vi "generate 96 well rois.vi"() -> ()   [LabVIEW 2013]
uses:
  <vilib>/vision/NI_Vision_Development_Module.lvlib
panel:
  in  "Save ROI data":path=path "C:/Users/Ed/Desktop/test temo2.png"
  out "roi data cluster":T1
  in  "Options":T2={"Interpolation Type"=enum."Bilinear Fixed", "Destination Width"=0, "Destination Height"=0, "Fill Value"=0.0}
  in  "Define Corner":bool
  in  "num Y cells":dbl=8.0
  in  "num X cells":dbl=12.0
  in  "three points":dbl[][](array[numeric])=[[86.0, 147.0], [2469.0, 46.0], [2531.0, 1640.0]]
  out "Image":T3(plugin-control)
  in  "Path to Image":path=path "C:/Users/Ed/Desktop/test temo2.png"
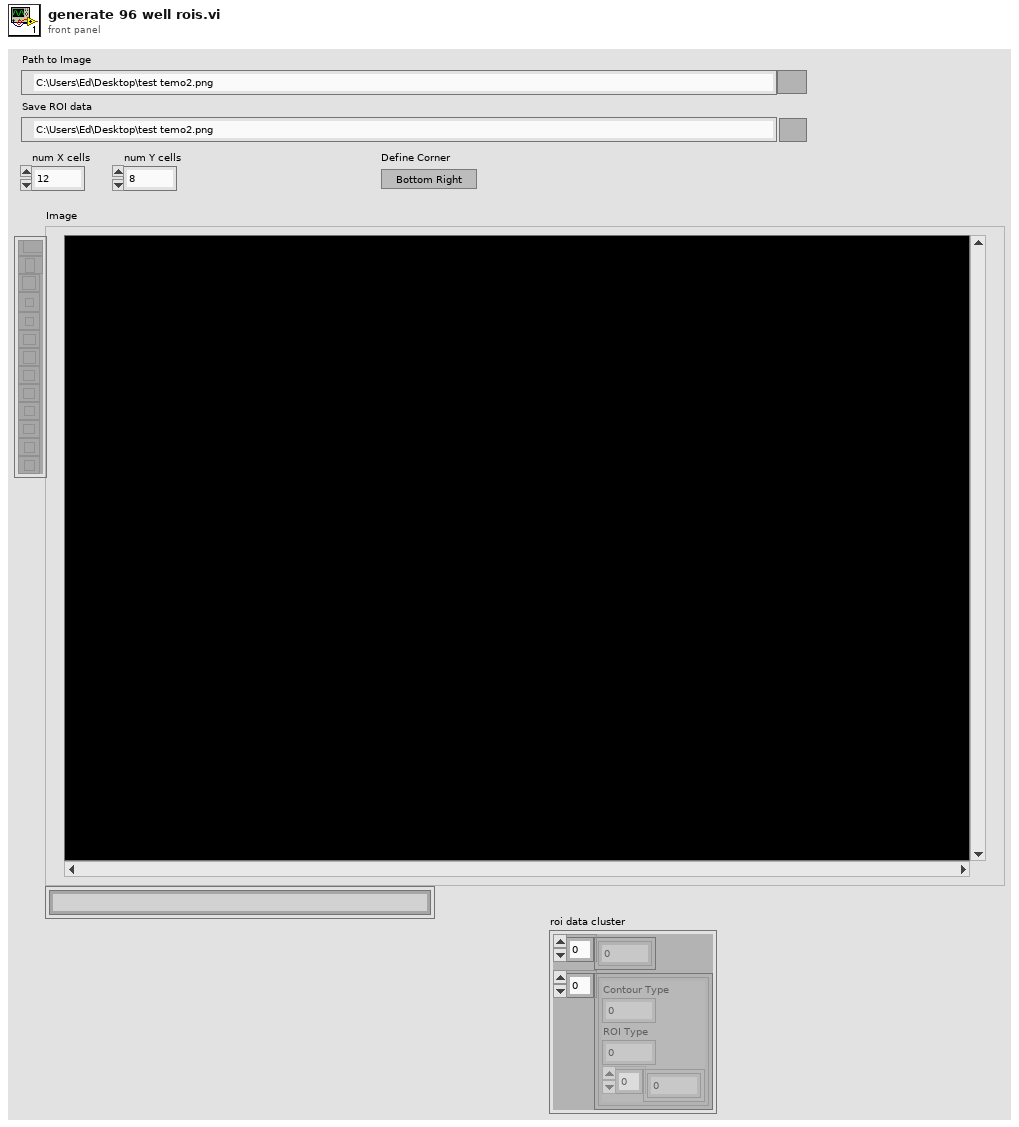
[diagram p1: front panel]
types:
  T1 = cluster{i32[], cluster{"Contour Type":u32, "ROI Type":u32, i32[]}[]}
  T2 = cluster{"Interpolation Type":enum32{"Zero Order", "Bilinear", "Quadratic", "Cubic", "Bilinear Fixed"}, "Destination Width":u32, "Destination Height":u32, "Fill Value":sgl}
  T3 = typedef "IMAQ Image.ctl" = refnum<image>
  T4 = enum16{"open", "replace", "create", "open or create", "replace or create", "replace or create with confirmation"}
  T5 = cluster{"Global Rectangle":i32[], "Contours":cluster{"Contour Type":u32, "ROI Type":u32, "Points":i32[]}[]}
  T6 = cluster{"Contour Type":u32, "ROI Type":u32, "Points":i32[]}[]
  T7 = cluster{"Contour Type":u32, "ROI Type":u32, "Points":i32[]}
  T8 = cluster{"Contour Type":u32, "ROI Type":u32, i32[]}
  T9 = cluster{"Contour Type":u32, "ROI Type":u32, i32[]}[]
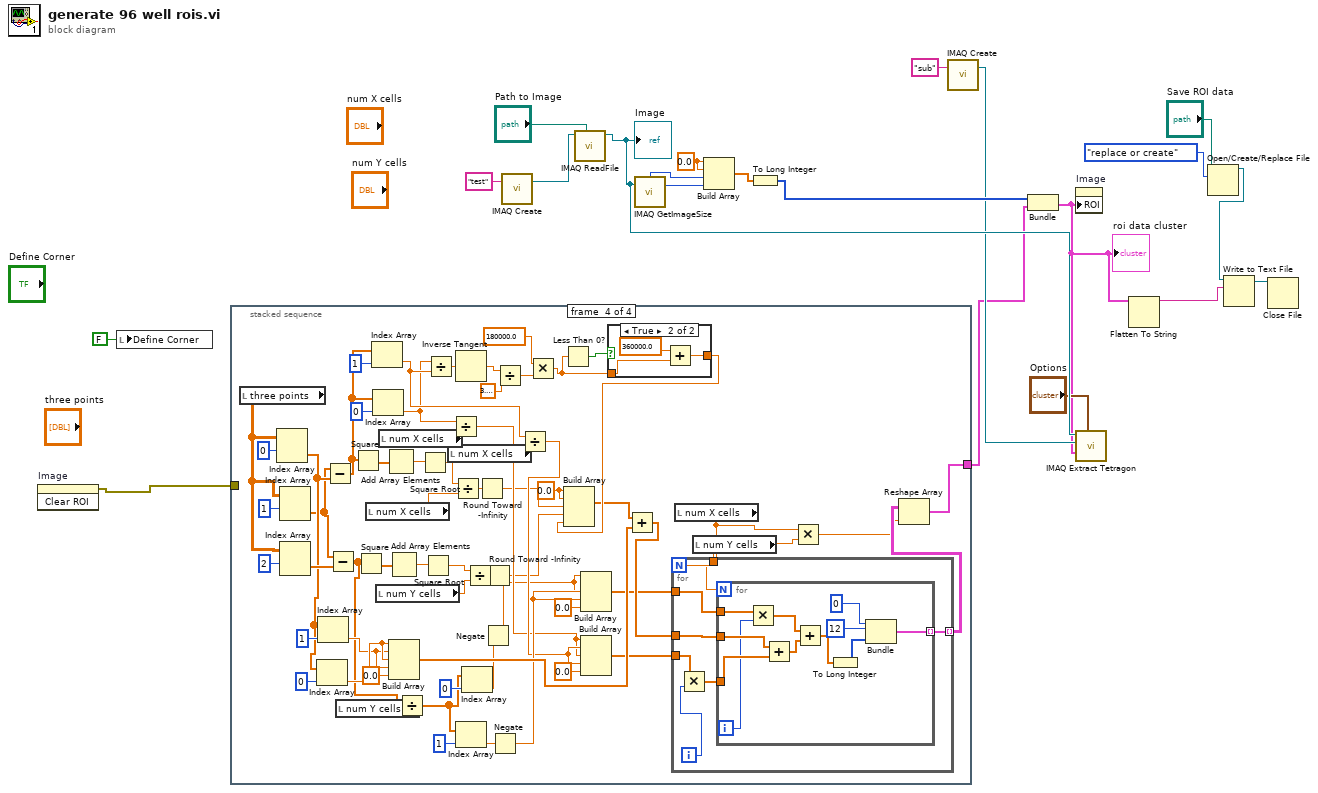
[diagram p0: block diagram]
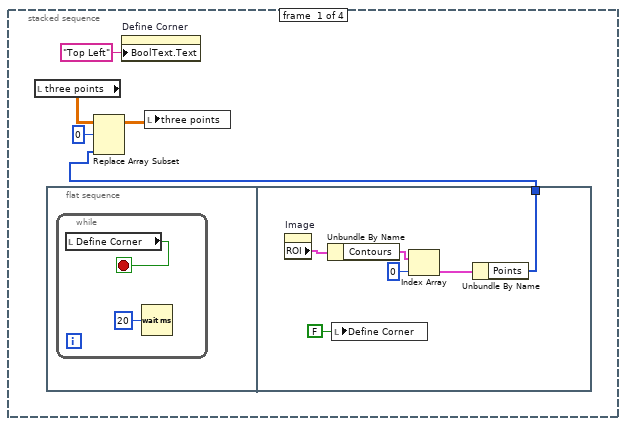
[diagram p2: hidden frame]
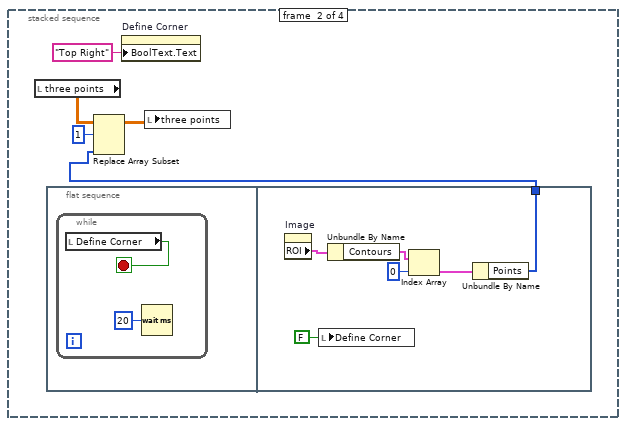
[diagram p3: hidden frame]
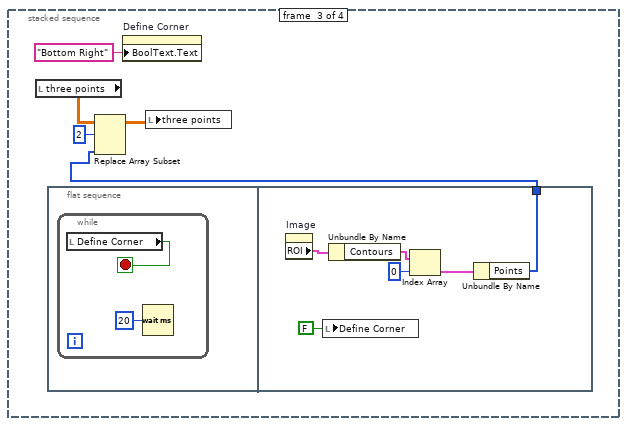
[diagram p4: hidden frame]
diagram:
  w17 = 0.0 ("element")
  n1 = invoke on="Image" class="ImageControl" method="Clear ROI"() -> (error out=w18:errorcluster)  [unwired: 3 in, 2 out]
  n2 = local write "Define Corner"(FALSE ("Define Corner")) -> ()
  n3 = stacked-sequence {
    tunnel: [_ _ _ w87] -> w7
    tunnel: w18 -> [_ _ _ _]
    frame #0 {
      n4 = local read "three points"() -> (w24:dbl[][])
      n5 = flat-sequence {
        tunnel: [w30] -> w25
        frame #0 {
          n6 = while {
            stop <- w28 stop-if-true
            n7 = local read "Define Corner"() -> (w28:bool)
            n8 = Wait (ms)(milliseconds to wait=u32 20) -> ()  [unwired: 1 out]
          }
        }
        frame #1 {
          n9 = property on="Image" class="ImageControl"() -> ("ROI"=w34:T5)  [unwired: 2 in, 2 out]
          n10 = Unbundle By Name(w34) -> ("Contours"=w33:T6)
          n11 = local write "Define Corner"(FALSE ("Define Corner")) -> ()
          n12 = Index Array(array=w33, index=0) -> (element=w31:T7)
          n13 = Unbundle By Name(w31) -> ("Points"=w30:i32[])
        }
      }
      n14 = Replace Array Subset(array=w24, new element=w25, index (row)=0) -> (w23:dbl[][])  [unwired: 1 in]
      n15 = property on="Define Corner" class="Bool (strict)"("BoolText.Text"="Top Left" ("Boolean Text.Text")) -> ()  [unwired: 2 in, 2 out]
      n16 = local write "three points"(w23) -> ()
    }
    frame #1 {
      n17 = local read "three points"() -> (w37:dbl[][])
      n18 = flat-sequence {
        tunnel: [w43] -> w38
        frame #0 {
          n19 = while {
            stop <- w41 stop-if-true
            n20 = local read "Define Corner"() -> (w41:bool)
            n21 = Wait (ms)(milliseconds to wait=u32 20) -> ()  [unwired: 1 out]
          }
        }
        frame #1 {
          n22 = property on="Image" class="ImageControl"() -> ("ROI"=w47:T5)  [unwired: 2 in, 2 out]
          n23 = local write "Define Corner"(FALSE ("Define Corner")) -> ()
          n24 = Unbundle By Name(w47) -> ("Contours"=w46:T6)
          n25 = Index Array(array=w46, index=0) -> (element=w44:T7)
          n26 = Unbundle By Name(w44) -> ("Points"=w43:i32[])
        }
      }
      n27 = Replace Array Subset(array=w37, new element=w38, index (row)=1) -> (w36:dbl[][])  [unwired: 1 in]
      n28 = property on="Define Corner" class="Bool (strict)"("BoolText.Text"="Top Right" ("Boolean Text.Text")) -> ()  [unwired: 2 in, 2 out]
      n29 = local write "three points"(w36) -> ()
    }
    frame #2 {
      n30 = local read "three points"() -> (w50:dbl[][])
      n31 = flat-sequence {
        tunnel: [w56] -> w51
        frame #0 {
          n32 = while {
            stop <- w54 stop-if-true
            n33 = local read "Define Corner"() -> (w54:bool)
            n34 = Wait (ms)(milliseconds to wait=u32 20) -> ()  [unwired: 1 out]
          }
        }
        frame #1 {
          n35 = property on="Image" class="ImageControl"() -> ("ROI"=w60:T5)  [unwired: 2 in, 2 out]
          n36 = local write "Define Corner"(FALSE ("Define Corner")) -> ()
          n37 = Unbundle By Name(w60) -> ("Contours"=w59:T6)
          n38 = Index Array(array=w59, index=0) -> (element=w57:T7)
          n39 = Unbundle By Name(w57) -> ("Points"=w56:i32[])
        }
      }
      n40 = Replace Array Subset(array=w50, new element=w51, index (row)=2) -> (w49:dbl[][])  [unwired: 1 in]
      n41 = property on="Define Corner" class="Bool (strict)"("BoolText.Text"="Bottom Right" ("Boolean Text.Text")) -> ()  [unwired: 2 in, 2 out]
      n42 = local write "three points"(w49) -> ()
    }
    frame #3 {
      w97 = 0.0 ("element")
      n43 = local read "three points"() -> (w68:dbl[][])
      n44 = Index Array(array=w68, index (row)=0) -> (element=w86:dbl[])  [unwired: 1 in]
      n45 = Index Array(array=w68, index (row)=1) -> (element=w85:dbl[])  [unwired: 1 in]
      n46 = Index Array(array=w68, index (row)=2) -> (element=w116:dbl[])  [unwired: 1 in]
      n47 = Index Array(array=w86, index=0) -> (element=w96:dbl)
      n48 = Index Array(array=w86, index=1) -> (element=w95:dbl)
      n49 = Subtract(x=w85, y=w86) -> (x-y=w109:dbl[])
      n50 = Subtract(x=w85, y=w116) -> (x-y=w82:dbl[])
      n51 = local read "num Y cells"() -> (w100:dbl)
      n52 = Square(x=w109) -> (x^2=w121:dbl[])
      n53 = Square(x=w82) -> (x^2=w117:dbl[])
      n54 = local read "num X cells"() -> (w115:dbl)
      n55 = Index Array(array=w109, index=1) -> (element=w66:dbl)
      n56 = Index Array(array=w109, index=0) -> (element=w65:dbl)
      n57 = local read "num Y cells"() -> (w113:dbl)
      n58 = local read "num X cells"() -> (w101:dbl)
      n59 = Add Array Elements(numeric array=w121) -> (sum=w120:dbl)
      n60 = Add Array Elements(numeric array=w117) -> (sum=w118:dbl)
      n61 = Build Array(w96, w95, w96, w95, 0.0 ("element")) -> (w93:dbl[])
      n62 = Divide(x=w82, y=w100) -> (x/y=w79:dbl[])
      n63 = Square Root(x=w120) -> (sqrt(x)=w102:dbl)
      n64 = Square Root(x=w118) -> (sqrt(x)=w114:dbl)
      n65 = Divide(x=w65, y=w66) -> (x/y=w69:dbl)
      n66 = local read "num X cells"() -> (w77:dbl)
      n67 = Divide(x=w65, y=w101) -> (x/y=w75:dbl)
      n68 = Divide(x=w102, y=w115) -> (x/y=w104:dbl)
      n69 = Inverse Tangent(1:w69) -> (0:w70:dbl)
      n70 = Index Array(array=w79, index=1) -> (element=w83:dbl)
      n71 = Index Array(array=w79, index=0) -> (element=w78:dbl)
      n72 = Divide(x=w114, y=w113) -> (x/y=w103:dbl)
      n73 = Round Toward -Infinity(1:w104) -> (0:w62:dbl)
      n74 = Negate(x=w78) -> (-x=w74:dbl)
      n75 = Round Toward -Infinity(1:w103) -> (0:w61:dbl)
      n76 = Negate(x=w83) -> (-x=w81:dbl)
      n77 = Divide(x=w70, y=3.141592653589793) -> (x/y=w67:dbl)
      n78 = Divide(x=w66, y=w77) -> (x/y=w76:dbl)
      n79 = Multiply(x=180000.0, y=w67) -> (x*y=w106:dbl)
      n80 = Less Than 0?(x=w106) -> (x < 0?=w107:bool)
      n81 = Build Array(w74, w81, w74, w81, 0.0 ("element")) -> (w89:dbl[])
      n82 = Build Array(w75, w76, w75, w76, 0.0 ("element")) -> (w90:dbl[])
      n83 = case shown="True" w107 {
        tunnel: w106 -> [w142 w144]
        tunnel: [w142 w143] -> w105
        frame False {
        }
        frame True {
          n84 = Add(x=360000.0, y=w144) -> (x+y=w143:dbl)
        }
      }
      n85 = Build Array(w97, w97, w62, w61, w105) -> (w92:dbl[])
      n86 = Add(x=w92, y=w93) -> (x+y=w91:dbl[])
      n87 = local read "num X cells"() -> (w73:dbl)
      n88 = local read "num Y cells"() -> (w72:dbl)
      n89 = for {
        N: w73 -> [_]
        tunnel: w72 -> [w130]
        tunnel: w91 -> [w129]
        tunnel: w90 -> [w127]
        tunnel: w89 -> [w128]
        tunnel: [w124] -> w88 mode=indexing
        i -> [w126]
        n90 = Multiply(x=w127, y=w126) -> (x*y=w125:dbl[])
        n91 = for {
          N: w130 -> [_]
          tunnel: w129 -> [w138]
          tunnel: w128 -> [w136]
          tunnel: w125 -> [w137]
          tunnel: [w131] -> w124 mode=indexing
          i -> [w135]
          n92 = Multiply(x=w136, y=w135) -> (x*y=w132:dbl[])
          n93 = Add(x=w138, y=w137) -> (x+y=w133:dbl[])
          n94 = Add(x=w132, y=w133) -> (x+y=w134:dbl[])
          n95 = To Long Integer(number=w134) -> (32bit integer=w139:i32[])
          n96 = Bundle("Contour Type"=u32 0, "ROI Type"=u32 12, w139) -> (w131:T8)  [unwired: 1 in]
        }
      }
      n97 = Multiply(x=w73, y=w72) -> (x*y=w71:dbl)
      n98 = Reshape Array(w88, w71) -> (w87:T9)
    }
  }
  n99 = call "IMAQ Create"("Image Name"="test") -> ("New Image"=w20:T3)  [unwired: 4 in, 1 out]
  n100 = call "IMAQ ReadFile"("File Path"="Path to Image", "Image"=w20) -> ("Image Out"=w10:T3)  [unwired: 5 in, 4 out]
  "Image" <- w10
  n101 = call "IMAQ GetImageSize"("Image"=w10) -> ("Y Resolution"=w15:i32, "X Resolution"=w16:i32)  [unwired: 3 in, 1 out]
  n102 = Build Array(w17, w17, w16, w15) -> (w14:dbl[])
  n103 = To Long Integer(number=w14) -> (32bit integer=w13:i32[])
  n104 = call "IMAQ Create"("Image Name"="sub") -> ("New Image"=w9:T3)  [unwired: 4 in, 1 out]
  n105 = Bundle(w13, w7) -> (w6:T1)  [unwired: 1 in]
  "roi data cluster" <- w6
  n106 = property on="Image" class="ImageControl"("ROI"=w6) -> ()  [unwired: 2 in, 2 out]
  n107 = call-poly "IMAQ Extract Tetragon"("Options"="Options", "ROI Descriptor"=w6, "Image Dst"=w9, "Image Src"=w10) -> ()  [unwired: 6 in, 2 out]
  n108 = Flatten To String(anything=w6) -> (data string=w2:string)  [unwired: 3 in, 2 out]
  n109 = Open/Create/Replace File(file path (use dialog)="Save ROI data", operation (0:open)=T4."replace or create") -> (refnum out=w3:refnum<file>)  [unwired: 4 in, 2 out]
  n110 = Write to Text File(file (use dialog)=w3, text=w2) -> (refnum out=w1:refnum<file>)  [unwired: 2 in, 2 out]
  n111 = Close File(refnum=w1) -> ()  [unwired: 1 in, 2 out]
